vi "week05_Ex02.vi"() -> ()   [LabVIEW 2017]
panel:
  out "Char 2":string
  out "number (0 to 1)  2":dbl
  out "round number (0 - 100) 2":u8
  out "Array":string[](array[string])
  out "Char":string
  out "round number (0 - 100)":u8
  out "number (0 to 1)":dbl
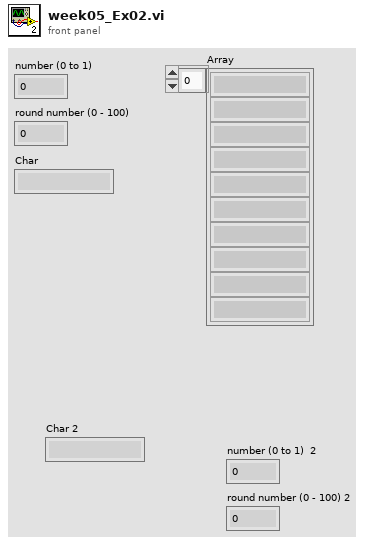
[diagram p1: front panel]
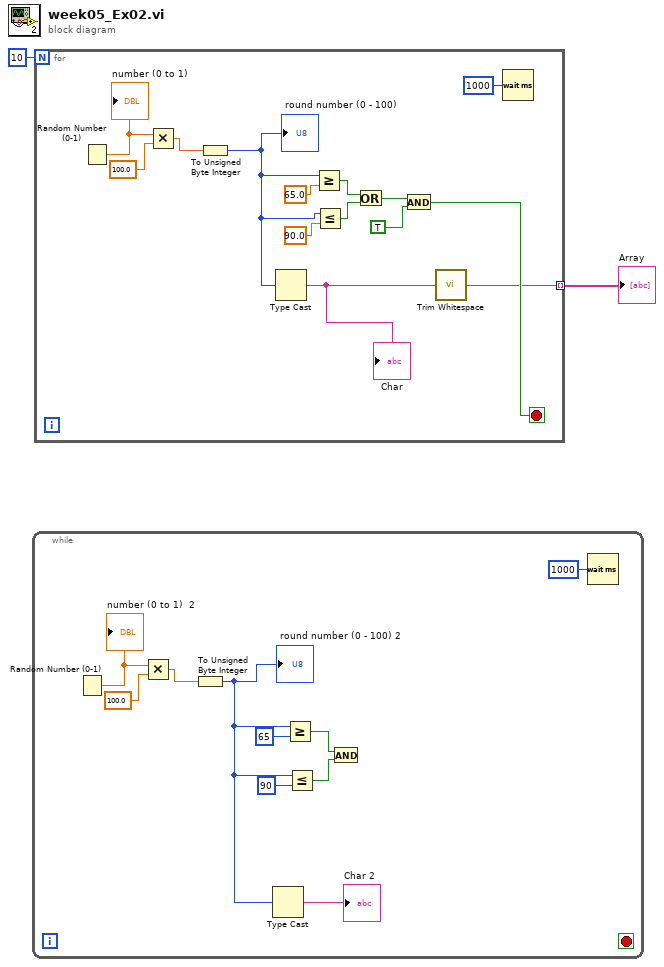
[diagram p0: block diagram]
diagram:
  n1 = while {
    stop <- _ stop-if-true
    n2 = Random Number (0-1)() -> (number: 0 to 1=w12:dbl)
    "number (0 to 1)  2" <- w12
    n3 = Multiply(x=w12, y=100.0) -> (x*y=w11:dbl)
    n4 = To Unsigned Byte Integer(number=w11) -> (unsigned 8bit integer=w6:u8)
    "round number (0 - 100) 2" <- w6
    n5 = Type Cast(x=w6) -> (*(type *) &x=→"Char 2":string)  [unwired: 1 in]
    n6 = Greater Or Equal?(x=w6, y=u8 65) -> (x >= y?=w3:bool)
    n7 = Less Or Equal?(x=w6, y=u8 90) -> (x <= y?=w4:bool)
    n8 = And(x=w3, y=w4) -> ()  [unwired: 1 out]
    n9 = Wait (ms)(milliseconds to wait=u32 1000) -> ()  [unwired: 1 out]
  }
  n10 = for {
    N: 10 -> [_]
    tunnel: [w13] -> w1 mode=indexing
    stop <- w15 stop-if-true
    n11 = Random Number (0-1)() -> (number: 0 to 1=w25:dbl)
    "number (0 to 1)" <- w25
    n12 = Multiply(x=w25, y=100.0) -> (x*y=w24:dbl)
    n13 = To Unsigned Byte Integer(number=w24) -> (unsigned 8bit integer=w20:u8)
    "round number (0 - 100)" <- w20
    n14 = Type Cast(x=w20) -> (*(type *) &x=w17:string)  [unwired: 1 in]
    "Char" <- w17
    n15 = Greater Or Equal?(x=w20, y=65.0) -> (x >= y?=w19:bool)
    n16 = Less Or Equal?(x=w20, y=90.0) -> (x <= y?=w18:bool)
    n17 = Or(x=w19, y=w18) -> (x .or. y?=w16:bool)
    n18 = And(x=w16, y=TRUE) -> (x .and. y?=w15:bool)
    n19 = call <vilib>:"Trim Whitespace.vi"("string"=w17) -> ("trimmed string"=w13:string)  [unwired: 1 in]
    n20 = Wait (ms)(milliseconds to wait=u32 1000) -> ()  [unwired: 1 out]
  }
  "Array" <- w1
